vi "M14_IR&Limits_Hardware_Begin.vi"   [LabVIEW 2019]
uses:
  <vilib>/Rock Robotics/SystemInterfaces/DIO/FPGA_DIOChannel.ctl
  M14_IR&Limits_Hardware_Globals.vi
types:
  T1 = typedef "FPGA_DIOChannel.ctl" = enum8{"DIO 0", "DIO 1", "DIO 2", "DIO 3", "DIO 4", "DIO 5", "DIO 6", "DIO 7", "DIO 8", "DIO 9", "DIO MXP 0", "DIO MXP 1", "DIO MXP 2", "DIO MXP 3", "DIO MXP 4", "DIO MXP 5", "DIO MXP 6", "DIO MXP 7", "DIO MXP 8", "DIO MXP 9", "DIO MXP 10", "DIO MXP 11", "DIO MXP 12", "DIO MXP 13", "DIO MXP 14", "DIO MXP 15", "SPI Port CS1", "SPI Port CS2", "SPI Port CS3", "SPI Port MISO", "SPI Port MOSI", "Invalid"}
  T2 = typedef "WPI_DigitalInputDevRef.ctl" = cluster{"DevStatus":errorcluster, "DIO Channel":T1}
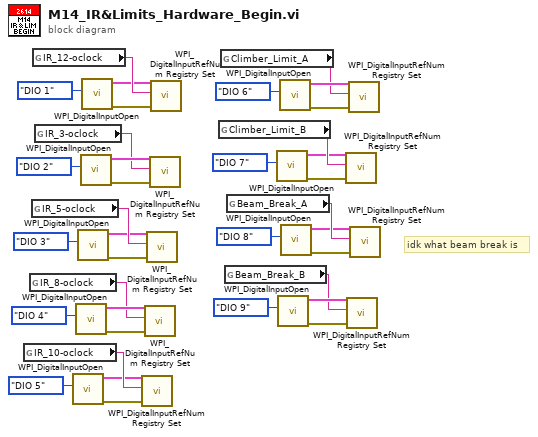
[diagram p0: block diagram]
diagram:
  # "idk what beam break is"
  n1 = global read "M14_IR&Limits_Hardware_Globals.vi" "IR_10-oclock"() -> (w28:string)
  n2 = global read "M14_IR&Limits_Hardware_Globals.vi" "IR_8-oclock"() -> (w21:string)
  n3 = global read "M14_IR&Limits_Hardware_Globals.vi" "IR_5-oclock"() -> (w20:string)
  n4 = global read "M14_IR&Limits_Hardware_Globals.vi" "IR_12-oclock"() -> (w12:string)
  n5 = global read "M14_IR&Limits_Hardware_Globals.vi" "IR_3-oclock"() -> (w13:string)
  n6 = call <vilib>:"WPI_DigitalInputOpen.vi"("DIO Channel"=FPGA_DIOChannel."DIO 5") -> ("error out"=w26:errorcluster, "DigitalInputDevRef"=w25:T2)  [unwired: 9 in]
  n7 = call <vilib>:"WPI_DigitalInputOpen.vi"("DIO Channel"=FPGA_DIOChannel."DIO 4") -> ("error out"=w23:errorcluster, "DigitalInputDevRef"=w24:T2)  [unwired: 9 in]
  n8 = call <vilib>:"WPI_DigitalInputOpen.vi"("DIO Channel"=FPGA_DIOChannel."DIO 3") -> ("error out"=w18:errorcluster, "DigitalInputDevRef"=w17:T2)  [unwired: 9 in]
  n9 = call <vilib>:"WPI_DigitalInputOpen.vi"("DIO Channel"=FPGA_DIOChannel."DIO 2") -> ("error out"=w15:errorcluster, "DigitalInputDevRef"=w16:T2)  [unwired: 9 in]
  n10 = call <vilib>:"WPI_DigitalInputOpen.vi"("DIO Channel"=FPGA_DIOChannel."DIO 1") -> ("error out"=w10:errorcluster, "DigitalInputDevRef"=w9:T2)  [unwired: 9 in]
  n11 = call <vilib>:"WPI_DigitalInputRefNum Registry Set.vi"("error in (no error)"=w26, "refnum name"=w28, "DigitalInputDevRef"=w25) -> ()  [unwired: 7 in, 2 out]
  n12 = call <vilib>:"WPI_DigitalInputRefNum Registry Set.vi"("error in (no error)"=w23, "refnum name"=w21, "DigitalInputDevRef"=w24) -> ()  [unwired: 7 in, 2 out]
  n13 = call <vilib>:"WPI_DigitalInputRefNum Registry Set.vi"("error in (no error)"=w18, "refnum name"=w20, "DigitalInputDevRef"=w17) -> ()  [unwired: 7 in, 2 out]
  n14 = call <vilib>:"WPI_DigitalInputRefNum Registry Set.vi"("error in (no error)"=w15, "refnum name"=w13, "DigitalInputDevRef"=w16) -> ()  [unwired: 7 in, 2 out]
  n15 = call <vilib>:"WPI_DigitalInputRefNum Registry Set.vi"("error in (no error)"=w10, "refnum name"=w12, "DigitalInputDevRef"=w9) -> ()  [unwired: 7 in, 2 out]
  n16 = global read "M14_IR&Limits_Hardware_Globals.vi" "Climber_Limit_B"() -> (w36:string)
  n17 = global read "M14_IR&Limits_Hardware_Globals.vi" "Climber_Limit_A"() -> (w29:string)
  n18 = global read "M14_IR&Limits_Hardware_Globals.vi" "Beam_Break_B"() -> (w1:string)
  n19 = global read "M14_IR&Limits_Hardware_Globals.vi" "Beam_Break_A"() -> (w8:string)
  n20 = call <vilib>:"WPI_DigitalInputOpen.vi"("DIO Channel"=FPGA_DIOChannel."DIO 7") -> ("error out"=w34:errorcluster, "DigitalInputDevRef"=w33:T2)  [unwired: 9 in]
  n21 = call <vilib>:"WPI_DigitalInputOpen.vi"("DIO Channel"=FPGA_DIOChannel."DIO 9") -> ("error out"=w3:errorcluster, "DigitalInputDevRef"=w4:T2)  [unwired: 9 in]
  n22 = call <vilib>:"WPI_DigitalInputOpen.vi"("DIO Channel"=FPGA_DIOChannel."DIO 6") -> ("error out"=w31:errorcluster, "DigitalInputDevRef"=w32:T2)  [unwired: 9 in]
  n23 = call <vilib>:"WPI_DigitalInputOpen.vi"("DIO Channel"=FPGA_DIOChannel."DIO 8") -> ("error out"=w6:errorcluster, "DigitalInputDevRef"=w5:T2)  [unwired: 9 in]
  n24 = call <vilib>:"WPI_DigitalInputRefNum Registry Set.vi"("error in (no error)"=w34, "refnum name"=w36, "DigitalInputDevRef"=w33) -> ()  [unwired: 7 in, 2 out]
  n25 = call <vilib>:"WPI_DigitalInputRefNum Registry Set.vi"("error in (no error)"=w3, "refnum name"=w1, "DigitalInputDevRef"=w4) -> ()  [unwired: 7 in, 2 out]
  n26 = call <vilib>:"WPI_DigitalInputRefNum Registry Set.vi"("error in (no error)"=w31, "refnum name"=w29, "DigitalInputDevRef"=w32) -> ()  [unwired: 7 in, 2 out]
  n27 = call <vilib>:"WPI_DigitalInputRefNum Registry Set.vi"("error in (no error)"=w6, "refnum name"=w8, "DigitalInputDevRef"=w5) -> ()  [unwired: 7 in, 2 out]
